vi "Check Trip Relay Task.vi"(8 "error in (no error)":errorcluster, 9 "Alarms":T1, 10 "Simulation Mode":string, 11 "task/channels in":refnum<k21>) -> (0 "error out":errorcluster, 3 "task out":refnum<k21>)   [LabVIEW 2026, in "Acquisition.lvlib"]
uses:
  Acquisition.lvlib
  Alarms.ctl
  <vilib>/DAQmx/write.llb/DAQmx Write (Digital Bool 1Line 1Point).vi
  <vilib>/DAQmx/miscellaneous.llb/DAQmx Fill In Error Info.vi
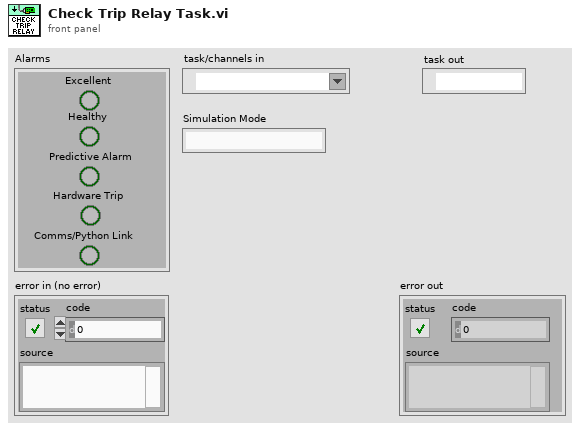
[diagram p1: front panel]
types:
  T1 = typedef "Alarms.ctl" = cluster{"Excellent":bool, "Healthy":bool, "Predictive Alarm":bool, "Hardware Trip":bool, "Comms/Python Link":bool}
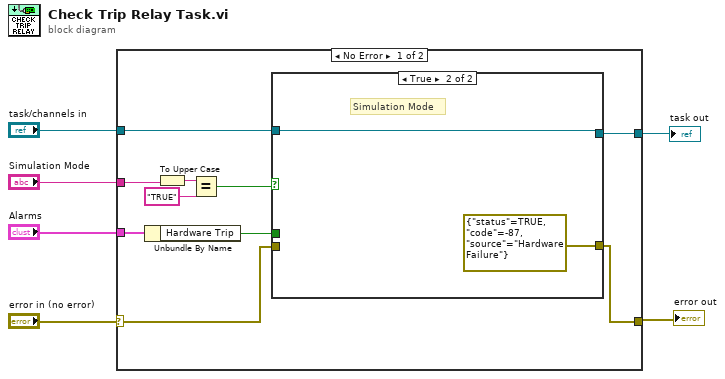
[diagram p0: block diagram]
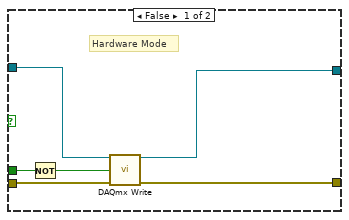
[diagram p2: hidden frame]
diagram:
  n1 = case shown="No Error" "error in (no error)" {
    selector: "error in (no error)" -> [w10 w26]
    tunnel: [w9 w26] -> w5
    tunnel: "Alarms" -> [w16 _]
    tunnel: "Simulation Mode" -> [w15 _]
    tunnel: [w7 w25] -> w1
    tunnel: "task/channels in" -> [w8 w25]
    frame No Error {
      n2 = Unbundle By Name(w16) -> ("Hardware Trip"=w11:bool)
      n3 = To Upper Case(1:w15) -> (0:w14:string)
      n4 = Equal?(x=w14, y="TRUE") -> (x = y?=w12:bool)
      n5 = case shown="True" w12 {
        tunnel: w11 -> [w22 _]
        tunnel: w10 -> [w20 _]
        tunnel: [w19 errorcluster {"status"=TRUE, "code"=-87, "source"="Hardware Failure"} ("error out")] -> w9
        tunnel: [w18 w24] -> w7
        tunnel: w8 -> [w17 w24]
        frame False {
          # "Hardware Mode"
          n6 = Not(x=w22) -> (.not. x?=w21:bool)
          n7 = call-poly <vilib>:"DAQmx Write.vi"("task/channels in"=w17, "data"=w21, "error in"=w20) -> ("task out"=w18:refnum<k21>, "error out"=w19:errorcluster)  [unwired: 10 in, 1 out]
        }
        frame True {
          # "Simulation Mode"
        }
      }
    }
    frame Error {
    }
  }
  "error out" <- w5
  "task out" <- w1
